vi "excel label to row and column.vi"(8 "error in (no error)":errorcluster, 11 "cell's name":string) -> (0 "error IO":errorcluster, 1 "output cluster":cluster{"row":i32, "column":i32}, 2 "column":i32, 3 "row":i32, 5 "Columns <255":bool)   [LabVIEW 2016]
uses:
  <vilib>/addons/_office/NI_ReportGenerationToolkit.lvlib
panel:
  out "cell's name 2":string
  out "match substring":string
  out "before substring":string
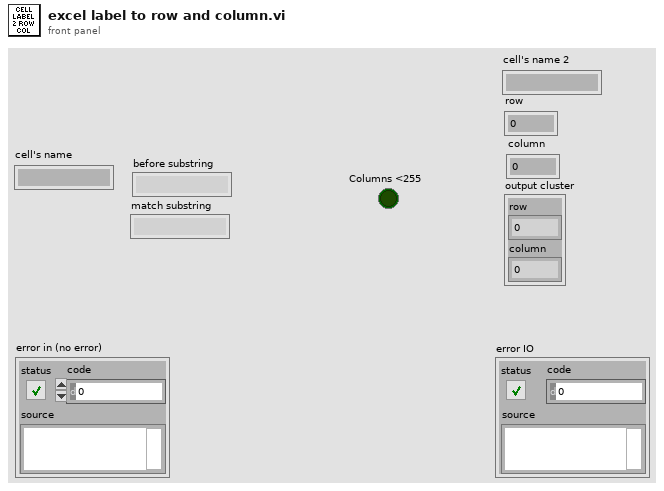
[diagram p1: front panel]
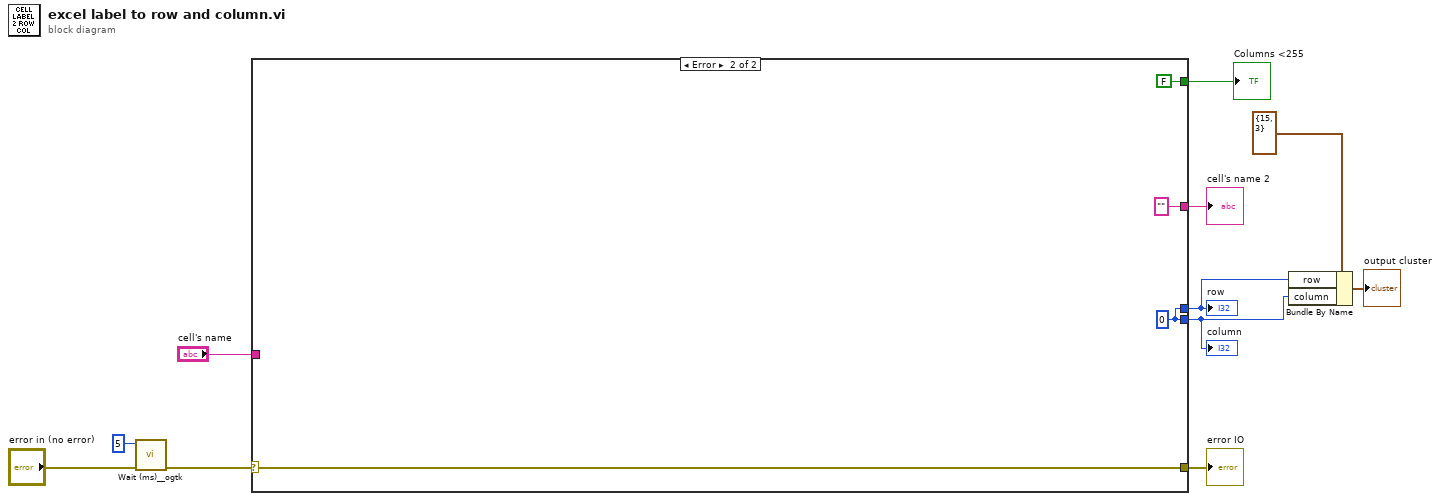
[diagram p0: block diagram]
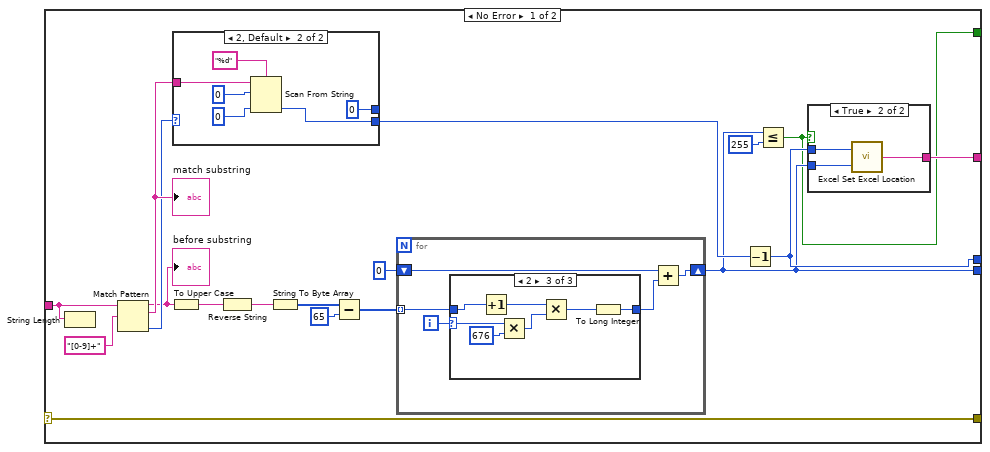
[diagram p2: hidden frame]
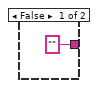
[diagram p3: hidden frame]
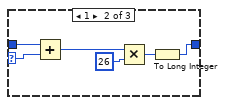
[diagram p5: hidden frame]
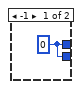
[diagram p6: hidden frame]
diagram:
  n1 = call "Wait (ms)__ogtk.vi"("error in (no error)"="error in (no error)", "milliseconds to wait"=u32 5) -> ("error out"=w3:errorcluster)  [unwired: 8 in, 1 out]
  n2 = case shown="Error" w3 {
    selector: w3 -> [w15 w63]
    tunnel: "cell's name" -> [w28 _]
    tunnel: [w22 "" ("cell's name")] -> w10
    tunnel: [w15 w63] -> w9
    tunnel: [w14 w62] -> w7
    tunnel: [w13 w62] -> w6
    tunnel: [w12 FALSE] -> w1
    frame No Error {
      n3 = String Length(string=w28) -> ()  [unwired: 1 out]
      n4 = Match Pattern(string=w28, regular expression="[0-9]+") -> (before substring=w24:string, match substring=w26:string, offset past match=w25:i32)  [unwired: 1 in, 1 out]
      "before substring" <- w24
      "match substring" <- w26
      n5 = To Upper Case(1:w24) -> (0:w19:string)
      n6 = case shown="2, Default" w25 {
        tunnel: [w53 w59] -> w29
        tunnel: w26 -> [_ w56]
        tunnel: [w53 0] -> _
        frame -1 {
          w53 = 0
        }
        frame 2, Default {
          n7 = Scan From String(format string="%d", input string=w56, initial scan location=u32 0, default 1=0) -> (output 1=w59:i32)  [unwired: 1 in, 3 out]
        }
      }
      n8 = Reverse String(1:w19) -> (0:w17:string)
      n9 = String To Byte Array(string=w17) -> (unsigned byte array=w23:u8[])
      n10 = Subtract(x=w23, y=u8 65) -> (x-y=w20:u8[])
      n11 = for {
        tunnel: w20 -> [w38] mode=indexing
        shift-right: [w34] -> w13
        shift-left: 0 -> [w36]
        i -> [w37]
        n12 = case shown="2" w37 {
          selector: w37 -> [_ w43 w46]
          tunnel: [w39 w45 w52] -> w35
          tunnel: w38 -> [w39 w41 w50]
          frame 0, Default {
          }
          frame 1 {
            n13 = Add(x=w41, y=w43) -> (x+y=w42:i32)
            n14 = Multiply(x=w42, y=26 ("x")) -> (x*y=w40:i32)
            n15 = To Long Integer(number=w40) -> (32bit integer=w45:i32)
          }
          frame 2 {
            n16 = Increment(x=w50) -> (x+1=w49:u8)
            n17 = Multiply(x=w46, y=676 ("x")) -> (x*y=w48:i32)
            n18 = Multiply(x=w49, y=w48) -> (x*y=w51:i32)
            n19 = To Long Integer(number=w51) -> (32bit integer=w52:i32)
          }
        }
        n20 = Add(x=w36, y=w35) -> (x+y=w34:i32)
      }
      n21 = Decrement(x=w29) -> (x-1=w14:i32)
      n22 = Less Or Equal?(x=w13, y=255 ("x")) -> (x <= y?=w12:bool)
      n23 = case shown="True" w12 {
        tunnel: ["" ("cell's name") w33] -> w22
        tunnel: w14 -> [_ w32]
        tunnel: w13 -> [_ w31]
        frame False {
        }
        frame True {
          n24 = call <vilib>:"Excel Set Excel Location.vi"("column"=w31, "row"=w32) -> ("cell's name"=w33:string)
        }
      }
    }
    frame Error {
      w62 = 0
    }
  }
  "cell's name 2" <- w10
  "error IO" <- w9
  "row" <- w7
  "column" <- w6
  "Columns <255" <- w1
  n25 = Bundle By Name(cluster=cluster{"row":i32, "column":i32} {"row"=15, "column"=3} ("start cell"), "row"=w7, "column"=w6) -> (→"output cluster":cluster{"row":i32, "column":i32})
